vi "interface_version.vi"(8 "error in (no error)":errorcluster, 11 "version in":T1) -> (0 "error out":errorcluster, 3 "version out":T1)   [LabVIEW 2015, in "lv-builder-default.lvlib"]
uses:
  lv-builder-default.lvlib
  public/_controls/version.ctl
  <vilib>/Utility/error.llb/Error Cluster From Error Code.vi
  <vilib>/ErrorRing/Error Ring.xnode
panel:
  out "version":string caption="Version"
  in  "fix":u32 caption="Fix"
  in  "minor":u32 caption="Minor"
  in  "major":u32 caption="Major"
  in  "suffix":string caption="Suffix"
  in  "cancel":bool
  in  "save":bool
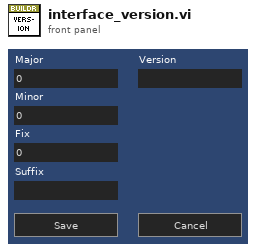
[diagram p1: front panel]
types:
  T1 = typedef "lv-builder-default.lvlib/version.ctl" = cluster{"project_file":string, "major":u32, "minor":u32, "fix":u32, "suffix":string}
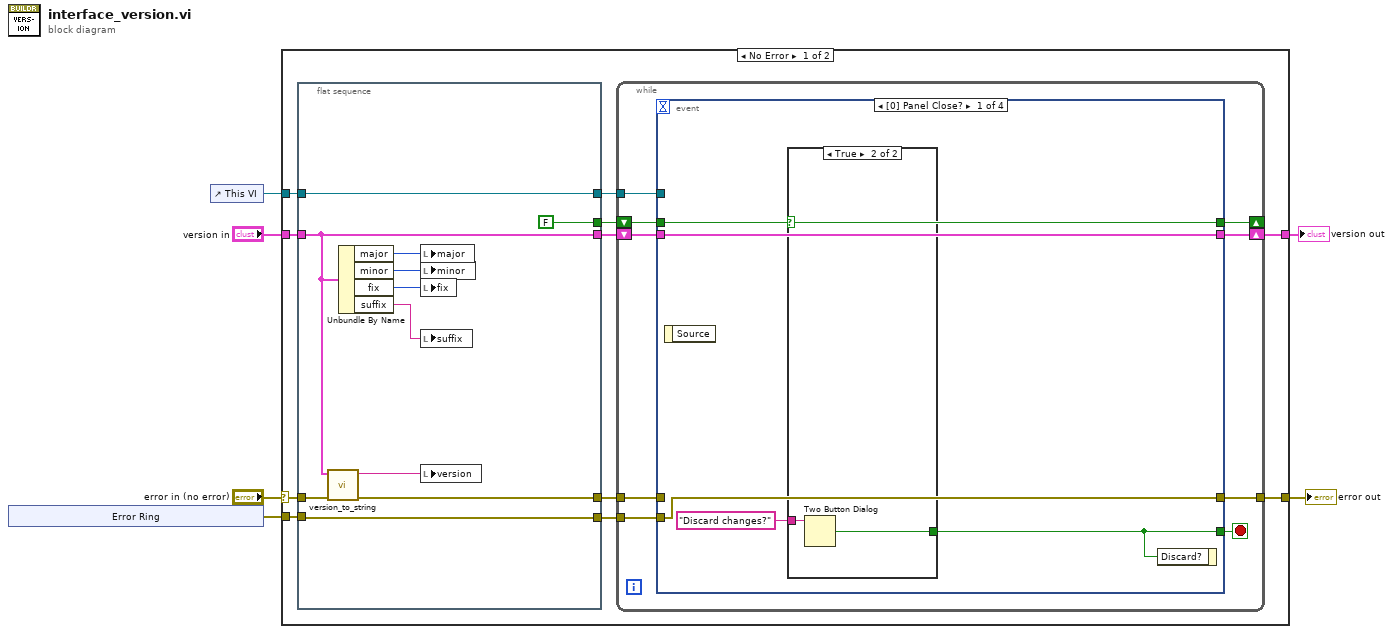
[diagram p0: block diagram]
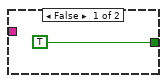
[diagram p2: hidden frame]
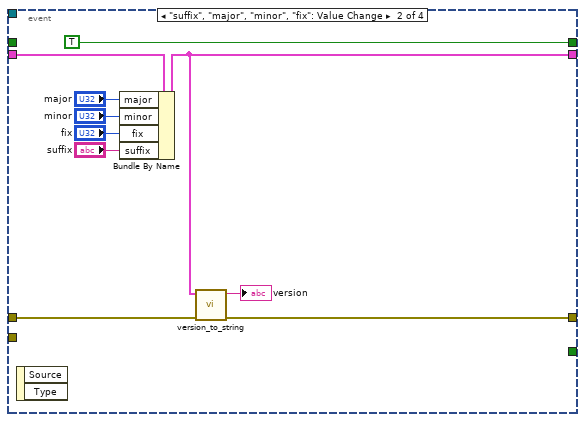
[diagram p3: hidden frame]
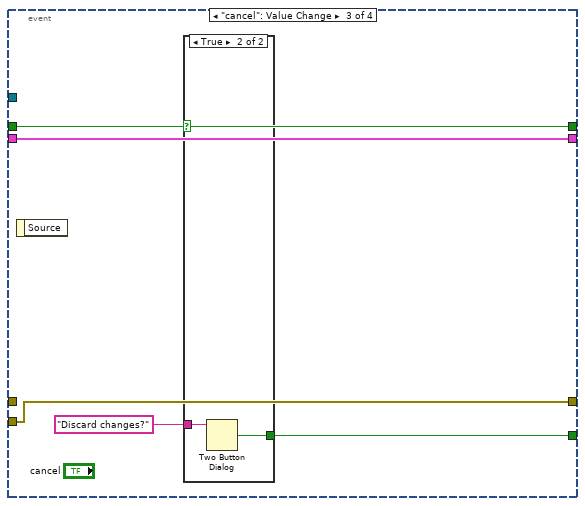
[diagram p4: hidden frame]
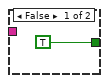
[diagram p5: hidden frame]
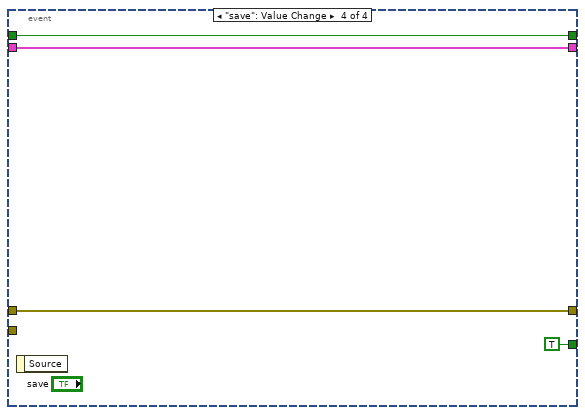
[diagram p6: hidden frame]
diagram:
  n1 = xnode "Error Ring"() -> ("error out"=w1:errorcluster)
  n2 = control-ref of="This VI"() -> (w4:refnum<vi>)
  n3 = case shown="No Error" "error in (no error)" {
    selector: "error in (no error)" -> [w17 w68]
    tunnel: [w11 w68] -> w5
    tunnel: w4 -> [w13 _]
    tunnel: [w10 _] -> w3
    tunnel: "version in" -> [w9 _]
    tunnel: w1 -> [w7 _]
    frame No Error {
      n4 = flat-sequence {
        tunnel: w17 -> [w20]
        tunnel: [w19] -> w16
        tunnel: [w21] -> w15
        tunnel: [w27] -> w14
        tunnel: w13 -> [w27]
        tunnel: [FALSE] -> w12
        tunnel: w9 -> [w21]
        tunnel: [w18] -> w8
        tunnel: w7 -> [w18]
        frame #0 {
          n5 = call "version_to_string.vi"("error in (no error)"=w20, "version"=w21) -> ("error out"=w19:errorcluster, "version"=w22:string)  [unwired: 8 in]
          n6 = Unbundle By Name(w21) -> ("major"=w26:u32, "minor"=w25:u32, "fix"=w24:u32, "suffix"=w23:string)
          n7 = local write "major"(w26) -> ()
          n8 = local write "minor"(w25) -> ()
          n9 = local write "fix"(w24) -> ()
          n10 = local write "suffix"(w23) -> ()
          n11 = local write "version"(w22) -> ()
        }
      }
      n12 = while {
        tunnel: w16 -> [w30]
        shift-right: [w35] -> w10
        shift-left: w15 -> [w36]
        tunnel: w14 -> [w32]
        shift-right: [w33] -> _
        shift-left: w12 -> [w34]
        tunnel: [w31] -> w11
        tunnel: w8 -> [w29]
        stop <- w37 stop-if-true
        n13 = event shown="[0] Panel Close?" {
          selector: _ -> [_ _ _ _]
          dyn-events: _ -> [_ _ _ _]
          timeout: _ -> [_ _ _ _]
          tunnel: [w40 _ w60 TRUE ("Discard?")] -> w37
          tunnel: w32 -> [_ _ _ _]
          tunnel: w36 -> [w42 w55 w59 w66]
          tunnel: [w42 w49 w59 w66] -> w35
          tunnel: w34 -> [w39 _ w57 w67]
          tunnel: [w39 TRUE w57 w67] -> w33
          tunnel: [w38 w46 w56 w65] -> w31
          tunnel: w30 -> [_ w47 _ w65]
          tunnel: w29 -> [w38 _ w56 _]
          event Panel Close? {
            n14 = event-data() -> ()  [unwired: 1 in, 1 out]
            n15 = case shown="True" w39 {
              tunnel: [TRUE ("Discard?") w45] -> w40
              tunnel: "Discard changes?" ("dialog_text") -> [_ w44]
              frame False {
              }
              frame True {
                n16 = Two Button Dialog(message=w44) -> (T button?=w45:bool)  [unwired: 2 in]
              }
            }
            n17 = event-data("Discard?"=w40) -> ()  [unwired: 1 in, 1 out]
          }
          event "suffix", "major", "minor", "fix": Value Change {
            n18 = event-data() -> ()  [unwired: 1 in, 2 out]
            n19 = Bundle By Name(cluster=w55, "major"="major", "minor"="minor", "fix"="fix", "suffix"="suffix") -> (w49:T1)
            n20 = call "version_to_string.vi"("error in (no error)"=w47, "version"=w49) -> ("error out"=w46:errorcluster, "version"=→"version":string)  [unwired: 8 in]
          }
          event "cancel": Value Change {
            n21 = event-data() -> ()  [unwired: 1 in, 1 out]
            n22 = case shown="True" w57 {
              tunnel: [TRUE ("Discard?") w62] -> w60
              tunnel: "Discard changes?" ("dialog_text") -> [_ w63]
              frame False {
              }
              frame True {
                n23 = Two Button Dialog(message=w63) -> (T button?=w62:bool)  [unwired: 2 in]
              }
            }
          }
          event "save": Value Change {
            n24 = event-data() -> ()  [unwired: 1 in, 1 out]
          }
        }
      }
    }
    frame Error {
    }
  }
  "error out" <- w5
  "version out" <- w3
